vi "set Property Value.vi"(6 "newValue":string, 7 "propertyName":string, 8 "error in":errorcluster, 9 "categoryName":string, 10 "resourceOrImageId":u32, 11 "cycloneHandle":u32) -> (0 "error out":errorcluster, 1 "categoryName out":string, 3 "function return":bool, 4 "newValue out":string, 5 "propertyName out":string)   [LabVIEW 2021, in "CycloneControlSDK.lvlib"]
doc: "extern \"C\" bool _cdecl setPropertyValue(uint32_t cycloneHandle, uint32_t resourceOrImageId, char *categoryName, char *propertyName, char *newValue);"
uses:
  CycloneControlSDK.lvlib
  CycloneControlSDK_64.dll
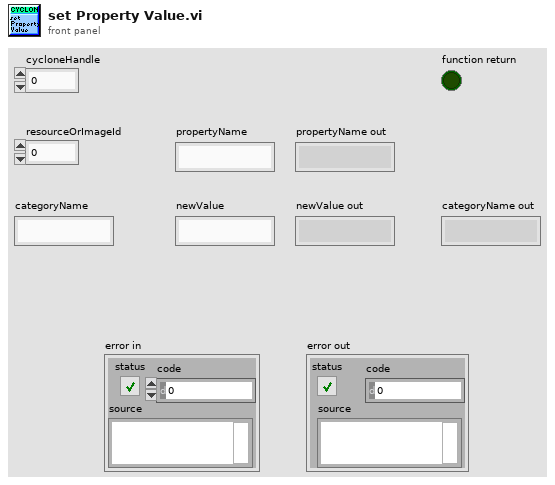
[diagram p1: front panel]
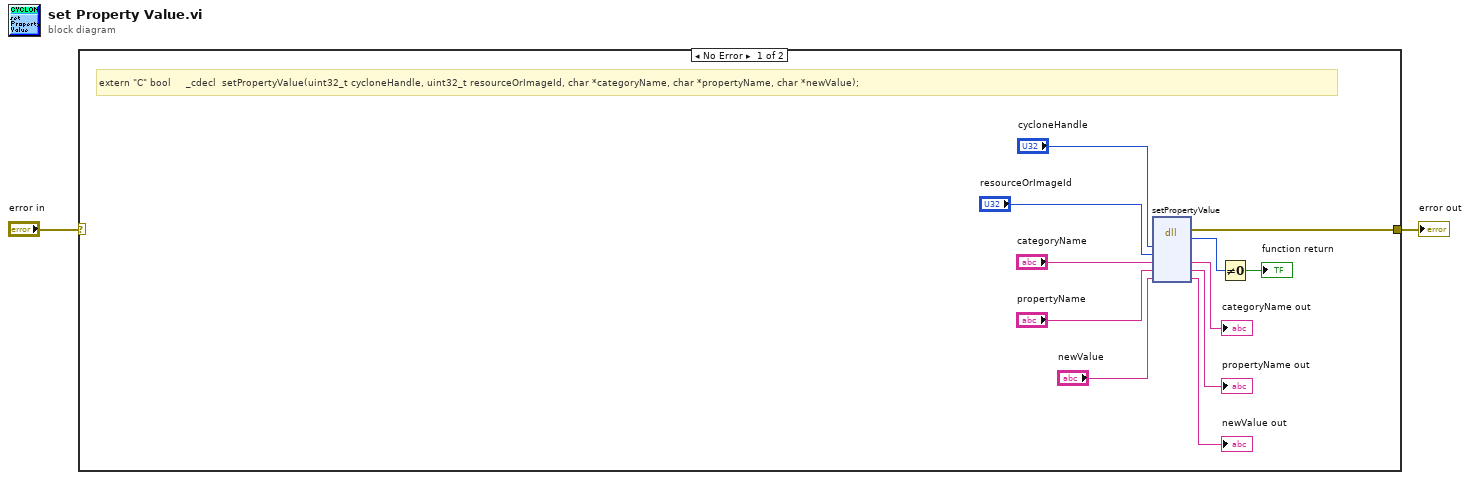
[diagram p0: block diagram]
diagram:
  n1 = case shown="No Error" "error in" {
    selector: "error in" -> [_ w14]
    tunnel: [w3 w14] -> w1
    frame No Error {
      # "extern \"C\" bool     _cdecl  setPropertyValue(uint32_t cycloneHandle, uint32_t resourceOrImageId, char *categoryName, char *propertyName, char *newValue);"
      n2 = dll-call lib="C:/PEMicro/cyclone/cycloneControl/controlsdk/examples/labview2018/user.lib/CycloneControlSDK/CycloneControlSDK_64.dll" fn="setPropertyValue"("cycloneHandle"="cycloneHandle", "resourceOrImageId"="resourceOrImageId", "categoryName"="categoryName", "propertyName"="propertyName", "newValue"="newValue") -> (error out=w3:errorcluster, "return type"=w12:u8, "categoryName"=→"categoryName out":string, "propertyName"=→"propertyName out":string, "newValue"=→"newValue out":string)  [unwired: 5 in, 1 out]
      n3 = Not Equal To 0?(x=w12) -> (x != 0?=→"function return":bool)
    }
    frame Error {
    }
  }
  "error out" <- w1
